vi "Set Variant Property.vi"(8 "error in (no error)":errorcluster, 10 "Property In":variant, 11 "2D Plot.lvclass":refnum<class "2D Plot.lvclass">) -> (0 "error out":errorcluster, 3 "2D Plot.lvclass":refnum<class "2D Plot.lvclass">)   [LabVIEW 2020, in "2D Plot.lvclass"]
uses:
  <vilib>/Math Plots/2D Math Plots/2D Plot/2D Plot/2D Plot.lvclass
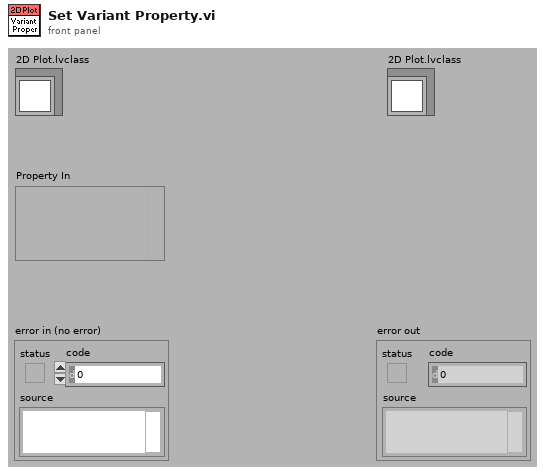
[diagram p1: front panel]
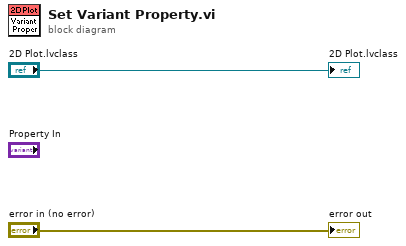
[diagram p0: block diagram]
diagram:
  "2D Plot.lvclass" <- "2D Plot.lvclass"
  "error out" <- "error in (no error)"
